vi "New UIConfiguration.vi"(8 "error in (no error)":errorcluster, 10 "Ini":path, 11 "UIConfiguration in":refnum<class "UIConfiguration.lvclass">) -> (0 "error out":errorcluster, 3 "UIConfiguration out":refnum<class "UIConfiguration.lvclass">)   [LabVIEW 2015, in "UIConfiguration.lvclass"]
uses:
  UIConfiguration.lvclass
  UIConfiguration.lvclass/UIConfiguration.ctl
  <vilib>/Utility/error.llb/Error Cluster From Error Code.vi
  <vilib>/ErrorRing/Error Ring.xnode
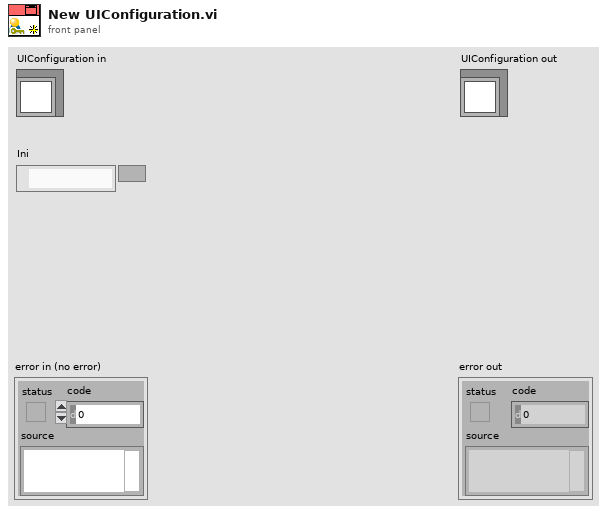
[diagram p1: front panel]
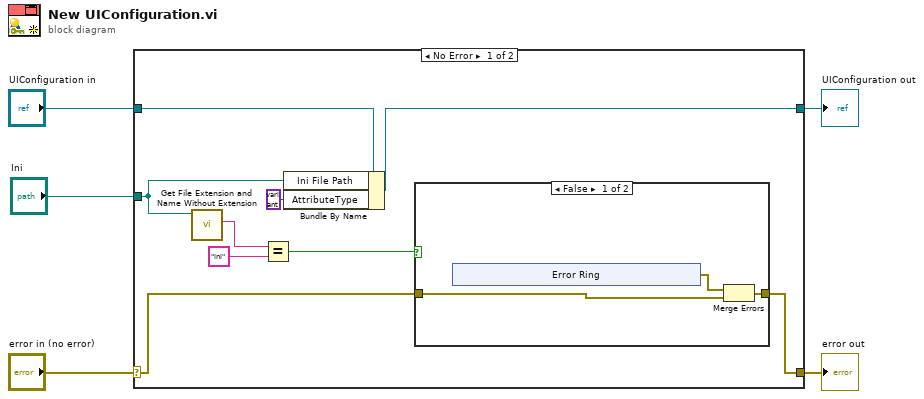
[diagram p0: block diagram]
diagram:
  n1 = case shown="No Error" "error in (no error)" {
    selector: "error in (no error)" -> [w11 w25]
    tunnel: [w10 w25] -> w4
    tunnel: [w6 w24] -> w2
    tunnel: "UIConfiguration in" -> [w9 w24]
    tunnel: "Ini" -> [w8 _]
    frame No Error {
      n2 = call <userlib>:"Get File Extension and Name Without Extension.vi"("file"=w8) -> ("lowercase file extension"=w14:string)  [unwired: 9 in, 1 out]
      n3 = Equal?(x=w14, y="ini") -> (x = y?=w12:bool)
      n4 = Bundle By Name(cluster=w9, "Ini File Path"=w8, "AttributeType"=variant ("Hashtable")) -> (w6:refnum<class "UIConfiguration.lvclass">)
      n5 = case shown="False" w12 {
        tunnel: w11 -> [w16 w23]
        tunnel: [w15 w23] -> w10
        frame False {
          n6 = xnode "Error Ring"() -> ("error out"=w17:errorcluster)
          n7 = Merge Errors(w17, w16) -> (w15:errorcluster)
        }
        frame True {
        }
      }
    }
    frame Error {
    }
  }
  "error out" <- w4
  "UIConfiguration out" <- w2
